vi "ICM Configuration Editor.vi"(11 "Inside a Program?":bool) -> ()   [LabVIEW 2018]
doc: "ICM Configuration Editor.vi\n\nThis Vi is a graphical configuration editor for ICM.\n\nInstrument Communication Module Version 1.0\nJuly, 2017 Original Code Consulting David Thomson\n www.originalcode.com"
uses:
  Controls/ICM Editor Tab.ctl
  Controls/ICM General Parameters.ctl
  Controls/ICM Config Editor State.ctl
  Controls/ICM Editor Command.ctl
  Scaling/Scaling Def.ctl
  Controls/ICM Config Command.ctl
  Query/Query.lvclass
  Scaling/Scaling.lvclass
  Scaling/Scaling.lvclass/Scaling.ctl
  Query/Query.lvclass/Query.ctl
  Query/Write Cycle Time (ms).vi
  Query/Read Cycle Time (ms).vi
  SubVIs/ICM Editor Stop.vi
  Parser/Parser.lvclass
panel:
  in  "File Loaded?":bool
  out "Config File":path
  in  "Stop":bool
  in  "Tab":T1
  in  "Save As":bool
  in  "Open/New":bool
  in  "Save":bool
  in  "Revert":bool
  in  "ICM General Parameters":T2 {"Time" format="%<%H:%M:%S>t"; "Date" format="%<%Y/%m/%d>T"; "Version" format="%.1g"}
  in  "Save Q":bool
  in  "Revert Q":bool
  in  "Cycle Time (ms)":u32
  in  "Queries":u16(ring) items=["Multiple Queries", "No Query", "Single Query"]
  in  "Bus":u16(ring) items=["Clock Time", "Modbus", "NI Analog", "Serial", "UDP"]
  in  "Parser":u16(ring) items=["General Parser", "Multi Sentence Parser", "No-op Parser", "Time Parser"]
  in  "Delete":bool
  in  "Add":bool
  in  "Instance":u16(ring) items=["(none)", "table", "hello", "hi"]
  in  "Save Scaling":bool
  in  "Revert Scaling":bool
  in  "Channel Scalings":i32(listbox)
  in  "Scaling":u16(ring) items=["Lookup Table", "Polynomial"]
  in  "Channel":u16(ring) items=["1", "Hour", "Minute", "Second", "Lat", "Long"]
  out "Error":errorcluster
  in  "Error Continue":bool
  in  "Error Quit":bool
  # "The values for these\nparameters are generally\nset by the ICM system and\nneed not be edited directly."
  # "Entries surrounded by \"***\" are present in the configuration file but\ndo not correspond to existing Channels, Scalings, or Instances."
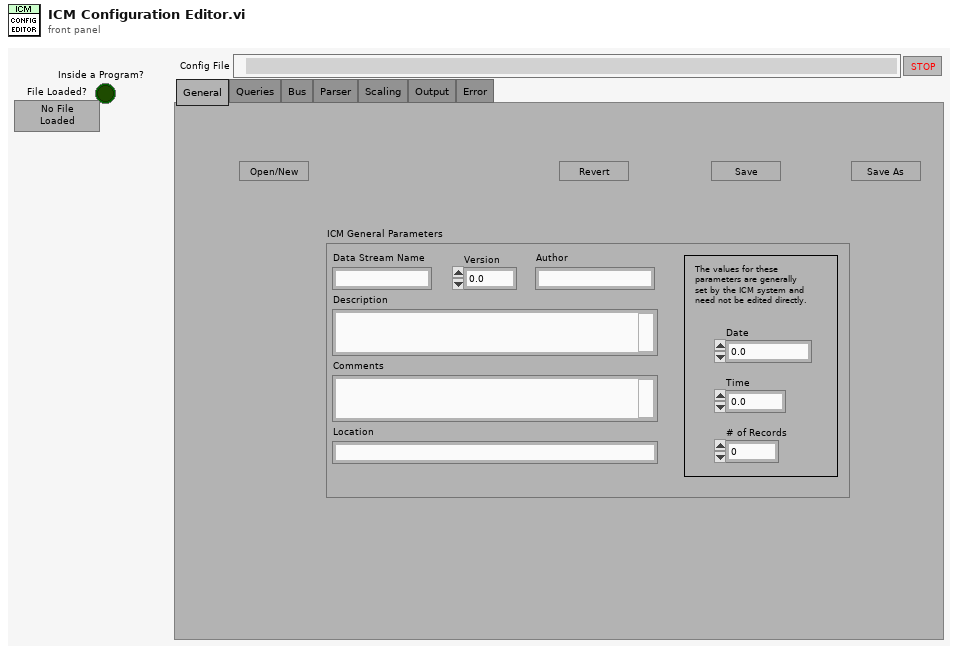
[diagram p1: front panel]
types:
  T1 = typedef "ICM Editor Tab.ctl" = enum32{"General", "Queries", "Bus", "Parser", "Scaling", "Output", "Error"}
  T2 = typedef "ICM General Parameters.ctl" = cluster{"Data Stream Name":string, "Version":sgl, "Author":string, "Description":string, "Comments":string, "Date":dbl, "Time":dbl, "Location":string, "# of Records":i32}
  T3 = typedef "ICM Config Editor State.ctl" = enum16{"Init", "Wait", "Read", "Write", "Load Queries", "Load Bus", "Load Parser", "Display Scaling", "Load Output", "Error", "Stop"}
  T4 = typedef "ICM Config Command.ctl" = enum16{"No-op", "Re-Display Sc."}
  T5 = typedef "ICM Editor Command.ctl" = enum16{"No-op", "Exit"}
  T6 = enum8{"Enabled", "Disabled", "Disabled and Grayed Out"}
  T7 = enum32{"Page Enabled", "Page Disabled", "Page Disabled & Grayed"}
  T8 = typedef "Scaling Def.ctl" = cluster{"Channel":string, "Scaling":string, "Instance":string}
  T9 = cluster{"Query.lvclass":refnum<class "Query.lvclass">, "ICM General Parameters":T2, "Config Queue":refnum<queue>, "Scaling Queue":refnum<queue>, "Query Queue":refnum<queue>, "Parser Queue":refnum<queue>, "Bus Queue":refnum<queue>, "Queries Loaded":bool, "Bus Loaded":bool, "Parser Loaded":bool, "Scaling Loaded":i32, "Instance Loaded":i32, "Scalings":T8[], "Flash?":bool}
  T10 = cluster{"RingText.Text":string, "RingText.Text":string, "RingText.Text":string}
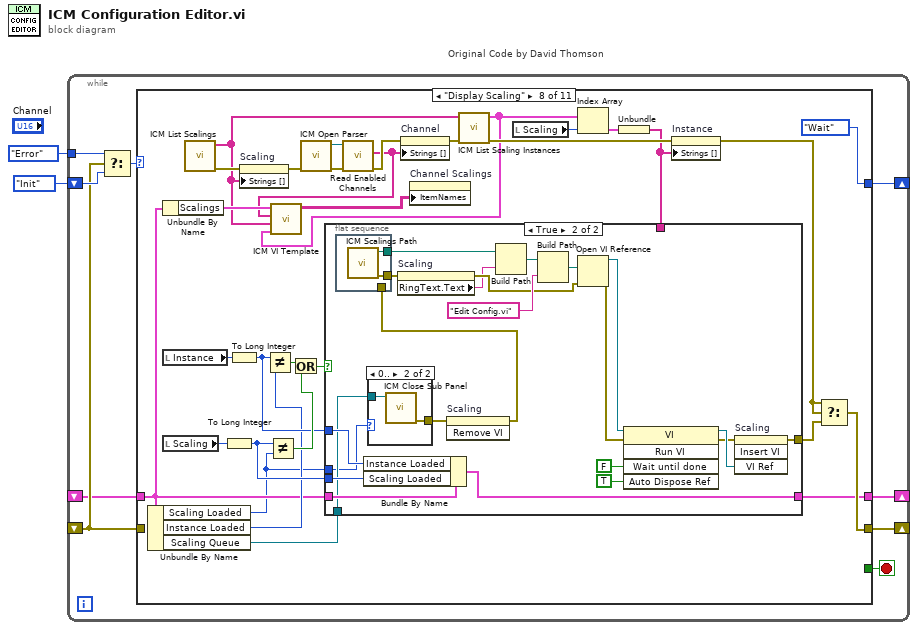
[diagram p0: block diagram]
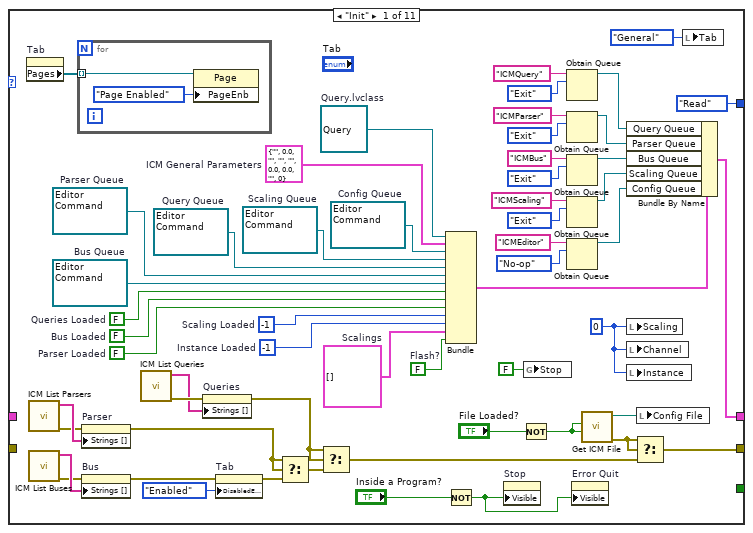
[diagram p2: hidden frame]
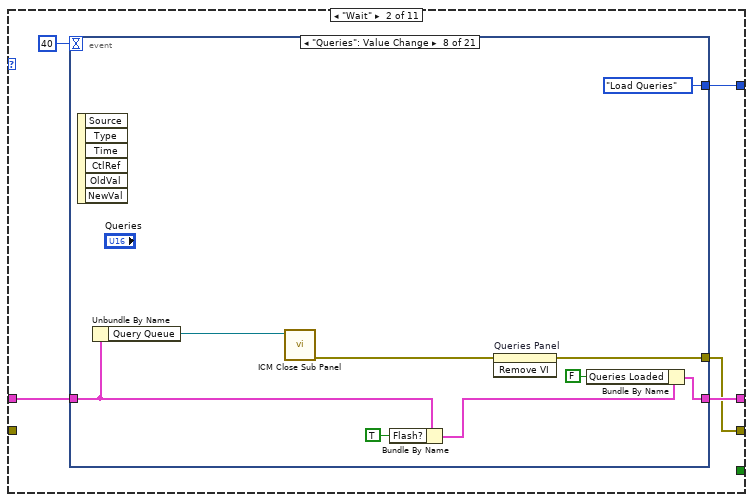
[diagram p3: hidden frame]
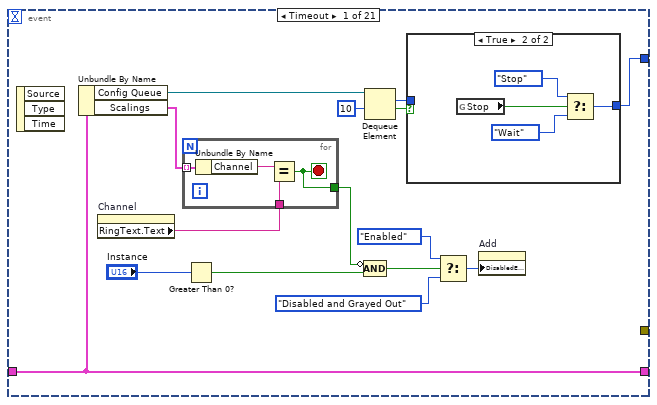
[diagram p4: hidden frame]
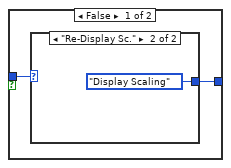
[diagram p5: hidden frame]
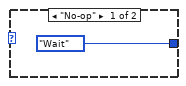
[diagram p6: hidden frame]
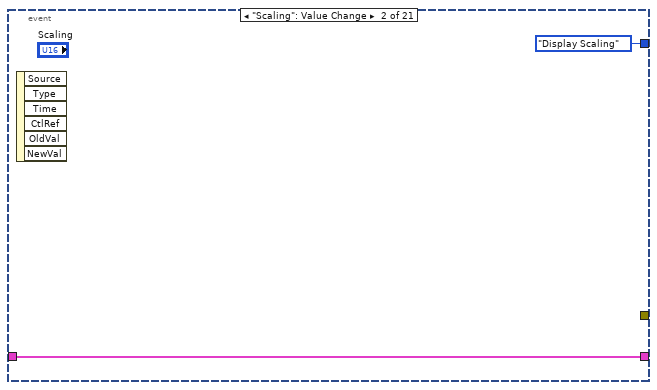
[diagram p7: hidden frame]
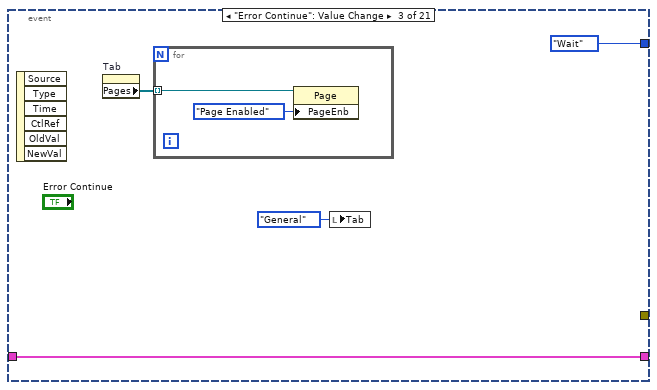
[diagram p8: hidden frame]
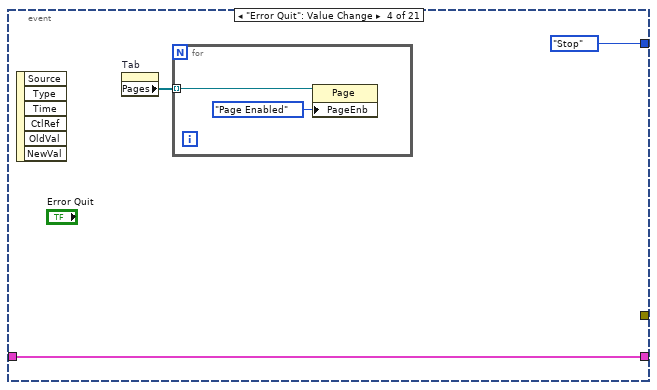
[diagram p9: hidden frame]
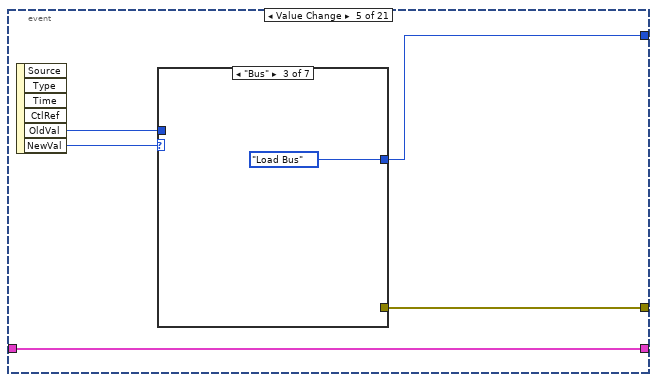
[diagram p10: hidden frame]
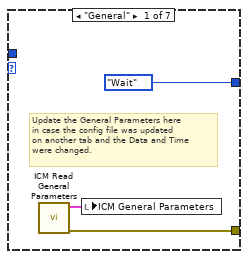
[diagram p11: hidden frame]
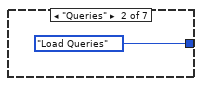
[diagram p12: hidden frame]
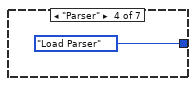
[diagram p13: hidden frame]
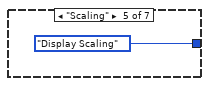
[diagram p14: hidden frame]
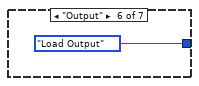
[diagram p15: hidden frame]
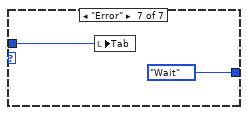
[diagram p16: hidden frame]
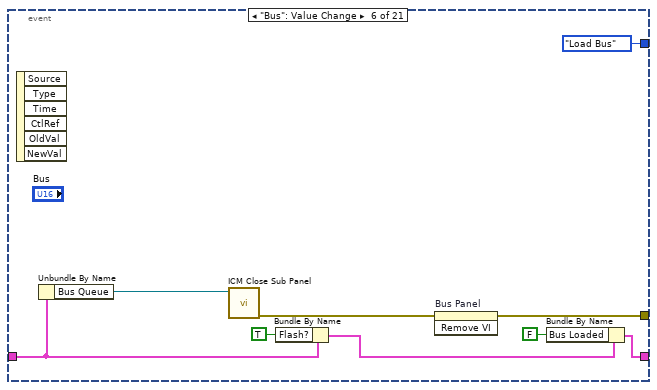
[diagram p17: hidden frame]
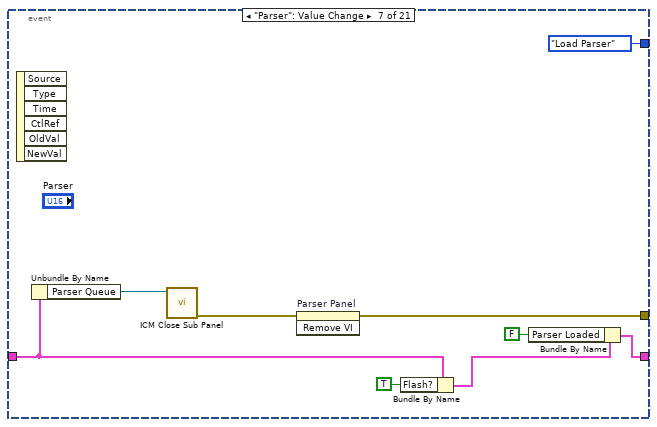
[diagram p18: hidden frame]
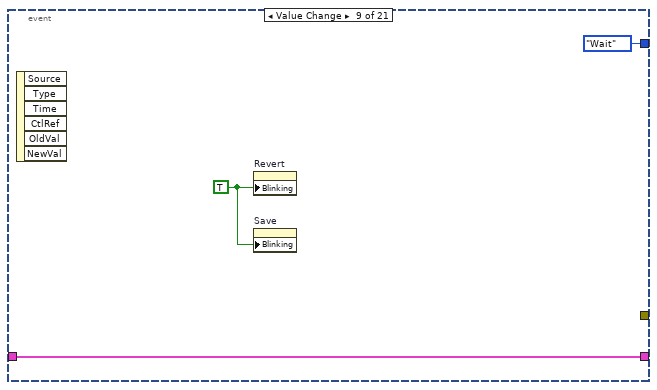
[diagram p19: hidden frame]
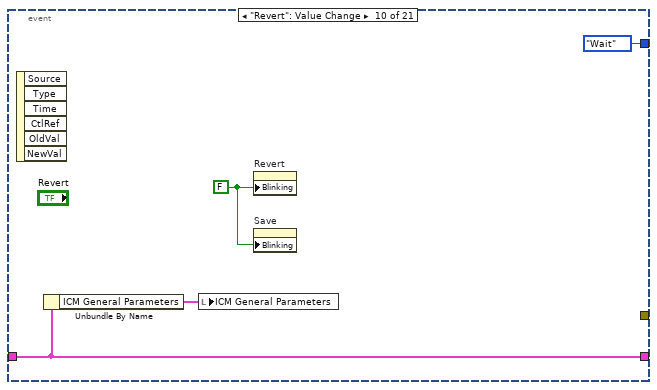
[diagram p20: hidden frame]
diagram:
  n1 = while "Original Code by David Thomson" {
    shift-right: [w5] -> _
    shift-left: ICM_Config_Editor_State."Init" ("Config State") -> [w9]
    shift-right: [w10] -> _
    shift-left: _ -> [w6]
    tunnel: ICM_Config_Editor_State."Error" ("Config State") -> [w7]
    shift-right: [w4] -> _
    shift-left: _ -> [w3]
    stop <- w11 stop-if-true
    n2 = Select(t=w7, s=w6, f=w9) -> (s? t:f=w8:T3)
    n3 = case shown="\"Display Scaling\"" w8 {
      tunnel: [_ _ _ _ _ _ _ _ _ _ TRUE] -> w11
      tunnel: [w60 w70 w261 w288 w297 w332 w361 w412 _ _ _] -> w10
      tunnel: w6 -> [_ _ _ _ _ _ _ _ _ w457 _]
      tunnel: [ICM_Config_Editor_State."Read" ("Config State") w73 ICM_Config_Editor_State."Wait" ("Config State") ICM_Config_Editor_State."Wait" ("Config State") ICM_Config_Editor_State."Wait" ("Config State") ICM_Config_Editor_State."Wait" ("Config State") ICM_Config_Editor_State."Write" ("Config State") ICM_Config_Editor_State."Wait" ("Config State") ICM_Config_Editor_State."Wait" ("Config State") ICM_Config_Editor_State."Wait" ("Config State") ICM_Config_Editor_State."Stop" ("Config State")] -> w5
      tunnel: [w53 w71 w277 w291 w293 w329 w362 w411 w452 w453 w486] -> w4
      tunnel: w3 -> [_ w72 w279 w291 w299 w330 w363 w398 w452 w453 w486]
      frame "Init" {
        w12 = FALSE  # Flash?
        w21 = refnum<class "Query.lvclass"> refnum  # Query.lvclass
        w23 = refnum<queue> refnum items=["No-op", "Re-Display Sc."]  # Config Queue
        w28 = refnum<queue> refnum items=["No-op", "Exit"]  # Scaling Queue
        w31 = u16 0
        w32 = -1  # Instance Loaded
        w34 = -1  # Scaling Loaded
        w33 = T8[] []  # Scalings
        w41 = refnum<queue> refnum items=["No-op", "Exit"]  # Query Queue
        w49 = refnum<queue> refnum items=["No-op", "Exit"]  # Parser Queue
        w50 = FALSE  # Parser Loaded
        w51 = FALSE  # Bus Loaded
        w52 = FALSE  # Queries Loaded
        w56 = refnum<queue> refnum items=["No-op", "Exit"]  # Bus Queue
        w24 = T2 {"Data Stream Name"="", "Version"=0.0, "Author"="", "Description"="", "Comments"="", "Date"=0.0, "Time"=0.0, "Location"="", "# of Records"=0}  # ICM General Parameters
        n4 = property on="Tab" class="TabCtl (strict)"() -> ("Pages"=w59:refnum<vi>[])  [unwired: 2 in, 2 out]
        n5 = call "ICM List Parsers.vi"() -> ("error out"=w45:errorcluster, "Parsers"=w46:string[])  [unwired: 10 in]
        n6 = call "ICM List Buses.vi"() -> ("error out"=w66:errorcluster, "Buses"=w67:string[])  [unwired: 10 in]
        n7 = for {
          tunnel: w59 -> [w69] mode=indexing
          n8 = property class="Page"(reference=w69, "PageEnb"=T7."Page Enabled" ("Page Enabled State")) -> ()  [unwired: 1 in, 2 out]
        }
        n9 = property on="Parser" class="Ring (strict)"(error in=w45, "Strings []"=w46) -> (error out=w43:errorcluster)  [unwired: 1 in, 1 out]
        n10 = property on="Bus" class="Ring (strict)"(error in=w66, "Strings []"=w67) -> (error out=w64:errorcluster)  [unwired: 1 in, 1 out]
        n11 = call "ICM List Queries.vi"() -> ("error out"=w39:errorcluster, "Queries"=w38:string[])  [unwired: 10 in]
        n12 = property on="Queries" class="Ring (strict)"(error in=w39, "Strings []"=w38) -> (error out=w36:errorcluster)  [unwired: 1 in, 1 out]
        n13 = property on="Tab" class="TabCtl (strict)"(error in=w64, "DisabledEnum"=T6."Enabled" ("Disabled")) -> (error out=w44:errorcluster)  [unwired: 1 in, 1 out]
        n14 = Select(t=w43, s=w43, f=w44) -> (s? t:f=w37:errorcluster)
        n15 = Select(t=w36, s=w36, f=w37) -> (s? t:f=w35:errorcluster)
        n16 = Bundle("Query.lvclass"=w21, "ICM General Parameters"=w24, "Config Queue"=w23, "Scaling Queue"=w28, "Query Queue"=w41, "Parser Queue"=w49, "Bus Queue"=w56, "Queries Loaded"=w52, "Bus Loaded"=w51, "Parser Loaded"=w50, "Scaling Loaded"=w34, "Instance Loaded"=w32, "Scalings"=w33, "Flash?"=w12) -> (w55:T9)  [unwired: 1 in]
        n17 = Not(x="Inside a Program?") -> (.not. x?=w14:bool)
        n18 = property on="Stop" class="Bool"("Visible"=w14) -> ()  [unwired: 2 in, 2 out]
        n19 = Not(x="File Loaded?") -> (.not. x?=w16:bool)
        n20 = global write "ICM Editor Stop.vi" "Stop"(FALSE ("Stop")) -> ()
        n21 = Obtain Queue(name (unnamed)="ICMQuery", element data type=ICM_Editor_Command."Exit" ("Editor Command")) -> (queue out=w40:refnum<queue>)  [unwired: 3 in, 2 out]
        n22 = Obtain Queue(name (unnamed)="ICMParser", element data type=ICM_Editor_Command."Exit" ("Editor Command")) -> (queue out=w47:refnum<queue>)  [unwired: 3 in, 2 out]
        n23 = Obtain Queue(name (unnamed)="ICMBus", element data type=ICM_Editor_Command."Exit" ("Editor Command")) -> (queue out=w54:refnum<queue>)  [unwired: 3 in, 2 out]
        n24 = Obtain Queue(name (unnamed)="ICMScaling", element data type=ICM_Editor_Command."Exit" ("Editor Command")) -> (queue out=w27:refnum<queue>)  [unwired: 3 in, 2 out]
        n25 = Obtain Queue(name (unnamed)="ICMEditor", element data type=ICM_Config_Command."No-op" ("Editor Command")) -> (queue out=w22:refnum<queue>)  [unwired: 3 in, 2 out]
        n26 = property on="Error Quit" class="Bool"("Visible"=w14) -> ()  [unwired: 2 in, 2 out]
        n27 = call "Get ICM File.vi"("Re-Init?"=w16, "Allow New?"=w16) -> ("error out"=w61:errorcluster, "ICM File"=w58:path)  [unwired: 8 in]
        n28 = Bundle By Name(cluster=w55, "Query Queue"=w40, "Parser Queue"=w47, "Bus Queue"=w54, "Scaling Queue"=w27, "Config Queue"=w22) -> (w53:T9)
        n29 = local write "Scaling"(w31) -> ()
        n30 = local write "Channel"(w31) -> ()
        n31 = local write "Instance"(w31) -> ()
        n32 = Select(t=w61, s=w61, f=w35) -> (s? t:f=w60:errorcluster)
        n33 = local write "Config File"(w58) -> ()
        n34 = local write "Tab"(ICM_Editor_Tab."General" ("Tab")) -> ()
      }
      frame "Wait" {
        n35 = event shown="[7] \"Queries\": Value Change" {
          selector: _ -> [_ _ _ _ _ _ _ _ _ _ _ _ _ _ _ _ _ _ _ _ _]
          dyn-events: _ -> [_ _ _ _ _ _ _ _ _ _ _ _ _ _ _ _ _ _ _ _ _]
          timeout: 40 -> [_ _ _ _ _ _ _ _ _ _ _ _ _ _ _ _ _ _ _ _ _]
          tunnel: [w85 ICM_Config_Editor_State."Display Scaling" ("Config State") ICM_Config_Editor_State."Wait" ("Config State") ICM_Config_Editor_State."Stop" ("Config State") w118 ICM_Config_Editor_State."Load Bus" ("Config State") ICM_Config_Editor_State."Load Parser" ("Config State") ICM_Config_Editor_State."Load Queries" ("Config State") ICM_Config_Editor_State."Wait" ("Config State") ICM_Config_Editor_State."Wait" ("Config State") ICM_Config_Editor_State."Write" ("Config State") ICM_Config_Editor_State."Read" ("Config State") w186 ICM_Config_Editor_State."Stop" ("Config State") ICM_Config_Editor_State."Display Scaling" ("Config State") ICM_Config_Editor_State."Display Scaling" ("Config State") ICM_Config_Editor_State."Wait" ("Config State") ICM_Config_Editor_State."Display Scaling" ("Config State") ICM_Config_Editor_State."Wait" ("Config State") ICM_Config_Editor_State."Wait" ("Config State") ICM_Config_Editor_State."Wait" ("Config State")] -> w73
          tunnel: w72 -> [w89 w103 w104 w110 w117 w131 w139 w148 w157 w161 w166 w171 w177 w200 w206 w222 w231 w236 w243 w252 w255]
          tunnel: [w89 w103 w104 w110 w117 w136 w146 w155 w157 w161 w164 w171 w185 w200 w205 w221 w231 w235 w243 w252 w255] -> w71
          tunnel: [_ _ _ _ w116 w137 w144 w153 _ _ _ _ w176 _ _ _ w227 w234 _ w247 w253] -> w70
          event Timeout {
            n36 = event-data() -> ()  [unwired: 1 in, 3 out]
            n37 = Unbundle By Name(w89) -> ("Config Queue"=w88:refnum<queue>, "Scalings"=w83:T8[])
            n38 = property on="Channel" class="Ring (strict)"() -> ("RingText.Text"=w82:string)  [unwired: 2 in, 2 out]
            n39 = for {
              tunnel: w83 -> [w91] mode=indexing
              tunnel: [w93] -> w81
              tunnel: w82 -> [w90]
              stop <- w93 stop-if-true
              n40 = Unbundle By Name(w91) -> ("Channel"=w92:string)
              n41 = Equal?(x=w92, y=w90) -> (x = y?=w93:bool)
            }
            n42 = Greater Than 0?(x="Instance") -> (x > 0?=w79:bool)
            n43 = Compound Arithmetic op=AND(invert w81, w79) -> (w76:bool)
            n44 = Dequeue Element(queue=w88, timeout in ms (-1)=10) -> (element=w84:T4, timed out?=w86:bool)  [unwired: 1 in, 2 out]
            n45 = case shown="True" w86 {
              tunnel: [w94 w101] -> w85
              tunnel: w84 -> [w95 _]
              frame False {
                n46 = case shown="\"Re-Display Sc.\"" w95 {
                  tunnel: [ICM_Config_Editor_State."Wait" ("Config State") ICM_Config_Editor_State."Display Scaling" ("Config State")] -> w94
                  frame "No-op" {
                  }
                  frame "Re-Display Sc." {
                  }
                }
              }
              frame True {
                n47 = global read "ICM Editor Stop.vi" "Stop"() -> (w100:bool)
                n48 = Select(t=ICM_Config_Editor_State."Stop" ("Config State"), s=w100, f=ICM_Config_Editor_State."Wait" ("Config State")) -> (s? t:f=w101:T3)
              }
            }
            n49 = Select(t=T6."Enabled" ("Disabled"), s=w76, f=T6."Disabled and Grayed Out" ("Disabled")) -> (s? t:f=w75:T6)
            n50 = property on="Add" class="Bool"("DisabledEnum"=w75) -> ()  [unwired: 2 in, 2 out]
          }
          event "Scaling": Value Change {
            n51 = event-data() -> ()  [unwired: 1 in, 6 out]
          }
          event "Error Continue": Value Change {
            n52 = event-data() -> ()  [unwired: 1 in, 6 out]
            n53 = property on="Tab" class="TabCtl (strict)"() -> ("Pages"=w105:refnum<vi>[])  [unwired: 2 in, 2 out]
            n54 = for {
              tunnel: w105 -> [w109] mode=indexing
              n55 = property class="Page"(reference=w109, "PageEnb"=T7."Page Enabled" ("Page Enabled State")) -> ()  [unwired: 1 in, 2 out]
            }
            n56 = local write "Tab"(ICM_Editor_Tab."General" ("Tab")) -> ()
          }
          event "Error Quit": Value Change {
            n57 = event-data() -> ()  [unwired: 1 in, 6 out]
            n58 = property on="Tab" class="TabCtl (strict)"() -> ("Pages"=w111:refnum<vi>[])  [unwired: 2 in, 2 out]
            n59 = for {
              tunnel: w111 -> [w114] mode=indexing
              n60 = property class="Page"(reference=w114, "PageEnb"=T7."Page Enabled" ("Page Enabled State")) -> ()  [unwired: 1 in, 2 out]
            }
          }
          event Value Change {
            n61 = event-data() -> ("OldVal"=w115:T1, "NewVal"=w119:T1)  [unwired: 1 in, 4 out]
            n62 = case shown="\"Bus\"" w119 {
              tunnel: [ICM_Config_Editor_State."Wait" ("Config State") ICM_Config_Editor_State."Load Queries" ("Config State") ICM_Config_Editor_State."Load Bus" ("Config State") ICM_Config_Editor_State."Load Parser" ("Config State") ICM_Config_Editor_State."Display Scaling" ("Config State") ICM_Config_Editor_State."Load Output" ("Config State") ICM_Config_Editor_State."Wait" ("Config State")] -> w118
              tunnel: [w120 _ _ _ _ _ _] -> w116
              tunnel: w115 -> [_ _ _ _ _ _ w128]
              frame "General" {
                # "Update the General Parameters here\nin case the config file was updated\non another tab and the Data and Time\nwere changed."
                n63 = call "ICM Read General Parameters.vi"() -> ("error out"=w120:errorcluster, "ICM General Parameters"=w121:T2)  [unwired: 7 in, 3 out]
                n64 = local write "ICM General Parameters"(w121) -> ()
              }
              frame "Queries" {
              }
              frame "Bus" {
              }
              frame "Parser" {
              }
              frame "Scaling" {
              }
              frame "Output" {
              }
              frame "Error" {
                n65 = local write "Tab"(w128) -> ()
              }
            }
          }
          event "Bus": Value Change {
            n66 = event-data() -> ()  [unwired: 1 in, 6 out]
            n67 = Unbundle By Name(w131) -> ("Bus Queue"=w134:refnum<queue>)
            n68 = call "ICM Close Sub Panel.vi"("Queue"=w134) -> ("error out"=w133:errorcluster)  [unwired: 9 in, 1 out]
            n69 = Bundle By Name(cluster=w131, "Flash?"=TRUE) -> (w132:T9)
            n70 = invoke on="Bus Panel" class="SubPnl" method="Remove VI"(error in=w133) -> (error out=w137:errorcluster)  [unwired: 2 in, 2 out]
            n71 = Bundle By Name(cluster=w132, "Bus Loaded"=FALSE) -> (w136:T9)
          }
          event "Parser": Value Change {
            n72 = event-data() -> ()  [unwired: 1 in, 6 out]
            n73 = Unbundle By Name(w139) -> ("Parser Queue"=w143:refnum<queue>)
            n74 = call "ICM Close Sub Panel.vi"("Queue"=w143) -> ("error out"=w142:errorcluster)  [unwired: 9 in, 1 out]
            n75 = invoke on="Parser Panel" class="SubPnl" method="Remove VI"(error in=w142) -> (error out=w144:errorcluster)  [unwired: 2 in, 2 out]
            n76 = Bundle By Name(cluster=w139, "Flash?"=TRUE) -> (w140:T9)
            n77 = Bundle By Name(cluster=w140, "Parser Loaded"=FALSE ("Bus Loaded")) -> (w146:T9)
          }
          event "Queries": Value Change {
            n78 = event-data() -> ()  [unwired: 1 in, 6 out]
            n79 = Unbundle By Name(w148) -> ("Query Queue"=w152:refnum<queue>)
            n80 = call "ICM Close Sub Panel.vi"("Queue"=w152) -> ("error out"=w151:errorcluster)  [unwired: 9 in, 1 out]
            n81 = Bundle By Name(cluster=w148, "Flash?"=TRUE) -> (w149:T9)
            n82 = invoke on="Queries Panel" class="SubPnl" method="Remove VI"(error in=w151) -> (error out=w153:errorcluster)  [unwired: 2 in, 2 out]
            n83 = Bundle By Name(cluster=w149, "Queries Loaded"=FALSE ("Bus Loaded")) -> (w155:T9)
          }
          event Value Change {
            w159 = TRUE ("Blinking")
            n84 = event-data() -> ()  [unwired: 1 in, 6 out]
            n85 = property on="Revert" class="Bool"("Blinking"=w159) -> ()  [unwired: 2 in, 2 out]
            n86 = property on="Save" class="Bool"("Blinking"=w159) -> ()  [unwired: 2 in, 2 out]
          }
          event "Revert": Value Change {
            w163 = FALSE ("Blinking")
            n87 = event-data() -> ()  [unwired: 1 in, 6 out]
            n88 = Unbundle By Name(w161) -> ("ICM General Parameters"=w160:T2)
            n89 = local write "ICM General Parameters"(w160) -> ()
            n90 = property on="Revert" class="Bool"("Blinking"=w163) -> ()  [unwired: 2 in, 2 out]
            n91 = property on="Save" class="Bool"("Blinking"=w163) -> ()  [unwired: 2 in, 2 out]
          }
          event "Save": Value Change {
            w168 = FALSE ("Blinking")
            n92 = event-data() -> ()  [unwired: 1 in, 6 out]
            n93 = property on="Revert" class="Bool"("Blinking"=w168) -> ()  [unwired: 2 in, 2 out]
            n94 = property on="Save" class="Bool"("Blinking"=w168) -> ()  [unwired: 2 in, 2 out]
            n95 = Bundle By Name(cluster=w166, "ICM General Parameters"="ICM General Parameters") -> (w164:T9)
          }
          event "Open/New": Value Change {
            w169 = TRUE ("Re-Init?")
            n96 = event-data() -> ()  [unwired: 1 in, 6 out]
            n97 = call "Get ICM File.vi"("Re-Init?"=w169, "Allow New?"=w169) -> ("ICM File"=→"Config File":path)  [unwired: 8 in, 1 out]
          }
          event "Save As": Value Change {
            n98 = event-data() -> ()  [unwired: 1 in, 6 out]
            n99 = call "Get ICM File.vi"() -> ("error out"=w179:errorcluster, "ICM File"=w178:path)  [unwired: 10 in]
            n100 = Strip Path(path=w178) -> (stripped path=w184:path)  [unwired: 1 out]
            n101 = call "File Dialog"("start path"=w184, "prompt"="Name the new configuration file:" ("pattern label"), "error in"=w179, "pattern (all files)"=".icm", "pattern label"="ICM Configuraiton File") -> ("selected path"=w180:path, "cancelled"=w174:bool, "error out"=w175:errorcluster)  [unwired: 7 in, 1 out]
            n102 = Compound Arithmetic op=AND(invert w174, invert w175) -> (w173:bool)
            n103 = case shown="True" w173 {
              tunnel: [ICM_Config_Editor_State."Wait" ("Config State") ICM_Config_Editor_State."Write" ("Config State")] -> w186
              tunnel: [w188 w190] -> w185
              tunnel: w180 -> [_ w195]
              tunnel: w178 -> [_ w197]
              tunnel: w177 -> [w188 w191]
              tunnel: [_ w192] -> w176
              frame False {
              }
              frame True {
                w198 = FALSE ("Blinking")
                n104 = Copy(9:TRUE ("overwrite (F)"), 10:w195, 11:w197) -> (0:w193:errorcluster)  [unwired: 2 in, 2 out]
                n105 = call "Get ICM File.vi"("ICM File In"=w195) -> ("error out"=w194:errorcluster)  [unwired: 9 in, 1 out]
                n106 = Select(t=w194, s=w194, f=w193) -> (s? t:f=w192:errorcluster)
                n107 = local read "ICM General Parameters"() -> (w189:T2)
                n108 = Bundle By Name(cluster=w191, "ICM General Parameters"=w189) -> (w190:T9)
                n109 = property on="Revert" class="Bool"("Blinking"=w198) -> ()  [unwired: 2 in, 2 out]
                n110 = property on="Save" class="Bool"("Blinking"=w198) -> ()  [unwired: 2 in, 2 out]
              }
            }
          }
          event "Stop": Value Change {
            n111 = event-data() -> ()  [unwired: 1 in, 6 out]
          }
          event "Add": Value Change {
            n112 = event-data() -> ()  [unwired: 1 in, 6 out]
            n113 = property on="Channel" class="Ring (strict)"() -> ("RingText.Text"=w204:string)  [unwired: 2 in, 2 out]
            n114 = property on="Scaling" class="Ring (strict)"() -> ("RingText.Text"=w210:string)  [unwired: 2 in, 2 out]
            n115 = property on="Instance" class="Ring (strict)"() -> ("RingText.Text"=w209:string)  [unwired: 2 in, 2 out]
            n116 = Unbundle By Name(w206) -> ("Scalings"=w203:T8[])
            n117 = Bundle("RingText.Text"=w204, "RingText.Text"=w210, "RingText.Text"=w209) -> (w208:T10)  [unwired: 1 in]
            n118 = for {
              tunnel: w204 -> [w213]
              tunnel: w203 -> [w215] mode=indexing
              tunnel: [w212] -> w202
              stop <- w212 stop-if-true
              n119 = Unbundle By Name(w215) -> ("Channel"=w214:string)
              n120 = Equal?(x=w213, y=w214) -> (x = y?=w212:bool)
            }
            n121 = case shown="False" w202 {
              tunnel: w208 -> [w218 _]
              tunnel: w203 -> [w217 w219]
              tunnel: [w216 w219] -> w207
              frame False {
                n122 = Build Array (concatenate)(w218, w217) -> (w216:T8[])
              }
              frame True {
              }
            }
            n123 = Bundle By Name(cluster=w206, "Scalings"=w207) -> (w205:T9)
          }
          event "Delete": Value Change {
            n124 = event-data() -> ()  [unwired: 1 in, 6 out]
            n125 = Unbundle By Name(w222) -> ("Scalings"=w225:T8[])
            n126 = Delete From Array(array=w225, length=1, index="Channel Scalings") -> (array with subset deleted=w223:T8[])  [unwired: 1 out]
            n127 = Bundle By Name(cluster=w222, "Scalings"=w223) -> (w221:T9)
          }
          event "Save Scaling": Value Change {
            n128 = event-data() -> ()  [unwired: 1 in, 6 out]
            n129 = Unbundle By Name(w231) -> ("Scalings"=w230:T8[])
            n130 = call "Write Scalings.vi"("Scalings"=w230, "Scaling in"=refnum<class "Scaling.lvclass"> refnum ("Scaling.lvclass")) -> ("error out"=w228:errorcluster, "Scaling out"=w229:refnum<class "Scaling.lvclass">)  [unwired: 8 in]
            n131 = call-dynamic "Write Config.vi"("error in (no error)"=w228, "Scaling in"=w229) -> ("error out"=w227:errorcluster)  [unwired: 8 in, 1 out]
          }
          event "Revert Scaling": Value Change {
            n132 = event-data() -> ()  [unwired: 1 in, 6 out]
            n133 = call-dynamic "Read Config.vi"("Scaling in"=refnum<class "Scaling.lvclass"> refnum ("Scaling.lvclass")) -> ("error out"=w239:errorcluster, "Scaling out"=w238:refnum<class "Scaling.lvclass">)  [unwired: 9 in]
            n134 = call "Read Scalings.vi"("error in (no error)"=w239, "Scaling in"=w238) -> ("error out"=w234:errorcluster, "Scalings"=w237:T8[])  [unwired: 7 in, 1 out]
            n135 = Bundle By Name(cluster=w236, "Scalings"=w237) -> (w235:T9)
          }
          event "Cycle Time (ms)": Value Change {
            w242 = TRUE ("Blinking")
            n136 = event-data() -> ()  [unwired: 1 in, 6 out]
            n137 = property on="Revert Q" class="Bool"("Blinking"=w242) -> ()  [unwired: 2 in, 2 out]
            n138 = property on="Save Q" class="Bool"("Blinking"=w242) -> ()  [unwired: 2 in, 2 out]
          }
          event "Save Q": Value Change {
            w245 = FALSE ("Blinking")
            n139 = event-data() -> ()  [unwired: 1 in, 6 out]
            n140 = Unbundle By Name(w252) -> ("Query.lvclass"=w251:refnum<class "Query.lvclass">)
            n141 = property class="Query.lvclass"(reference=w251, "Properties:Cycle Time (ms)"="Cycle Time (ms)") -> (reference out=w249:refnum<class "Query.lvclass">, error out=w248:errorcluster)  [unwired: 1 in]
            n142 = call-dynamic "Write Config.vi"("error in (no error)"=w248, "Query in"=w249) -> ("error out"=w247:errorcluster)  [unwired: 8 in, 1 out]
            n143 = property on="Revert Q" class="Bool"("Blinking"=w245) -> ()  [unwired: 2 in, 2 out]
            n144 = property on="Save Q" class="Bool"("Blinking"=w245) -> ()  [unwired: 2 in, 2 out]
          }
          event "Revert Q": Value Change {
            w258 = FALSE ("Blinking")
            n145 = event-data() -> ()  [unwired: 1 in, 6 out]
            n146 = property on="Revert Q" class="Bool"("Blinking"=w258) -> ()  [unwired: 2 in, 2 out]
            n147 = property on="Save Q" class="Bool"("Blinking"=w258) -> ()  [unwired: 2 in, 2 out]
            n148 = Unbundle By Name(w255) -> ("Query.lvclass"=w256:refnum<class "Query.lvclass">)
            n149 = property class="Query.lvclass"(reference=w256) -> (error out=w253:errorcluster, "Properties:Cycle Time (ms)"=w254:u32)  [unwired: 1 in, 1 out]
            n150 = local write "Cycle Time (ms)"(w254) -> ()
          }
        }
      }
      frame "Read" {
        n151 = property on="Queries" class="Ring (strict)"() -> ("Strings []"=w267:string[])  [unwired: 2 in, 2 out]
        n152 = property on="Bus" class="Ring (strict)"() -> ("Strings []"=w284:string[])  [unwired: 2 in, 2 out]
        n153 = property on="Parser" class="Ring (strict)"() -> ("Strings []"=w271:string[])  [unwired: 2 in, 2 out]
        n154 = call "ICM Read General Parameters.vi"() -> ("error out"=w264:errorcluster, "Parser"=w273:string, "Bus"=w285:string, "ICM General Parameters"=w278:T2, "Query"=w265:string)  [unwired: 7 in]
        n155 = Search 1D Array(1D array=w284, element=w285) -> (index of element=w282:i32)  [unwired: 1 in]
        n156 = Search 1D Array(1D array=w271, element=w273) -> (index of element=w275:i32)  [unwired: 1 in]
        n157 = Search 1D Array(1D array=w267, element=w265) -> (index of element=w270:i32)  [unwired: 1 in]
        n158 = Less Than 0?(x=w282) -> (x < 0?=w283:bool)
        n159 = Less Than 0?(x=w275) -> (x < 0?=w274:bool)
        n160 = Less Than 0?(x=w270) -> (x < 0?=w269:bool)
        n161 = call-dynamic "Read Config.vi"("error in (no error)"=w264, "Scaling in"=refnum<class "Scaling.lvclass"> refnum ("Scaling.lvclass")) -> ("error out"=w262:errorcluster, "Scaling out"=w260:refnum<class "Scaling.lvclass">)  [unwired: 8 in]
        n162 = Select(t=0, s=w283, f=w282) -> (s? t:f=w280:i32)
        n163 = Select(t=0, s=w274, f=w275) -> (s? t:f=w272:i32)
        n164 = Select(t=0, s=w269, f=w270) -> (s? t:f=w266:i32)
        n165 = local write "Queries"(w266) -> ()
        n166 = local write "Bus"(w280) -> ()
        n167 = local write "Parser"(w272) -> ()
        n168 = call "Read Scalings.vi"("error in (no error)"=w262, "Scaling in"=w260) -> ("error out"=w261:errorcluster, "Scalings"=w259:T8[])  [unwired: 7 in, 1 out]
        n169 = local write "ICM General Parameters"(w278) -> ()
        n170 = Bundle By Name(cluster=w279, "ICM General Parameters"=w278, "Scalings"=w259) -> (w277:T9)
      }
      frame "Write" {
        n171 = Unbundle By Name(w291) -> ("ICM General Parameters"=w290:T2)
        n172 = call "ICM Write General Parameters.vi"("ICM General Parameters"=w290) -> ("error out"=w289:errorcluster)  [unwired: 10 in]
        n173 = call "ICM Update Date and Time.vi"("error in (no error)"=w289) -> ("error out"=w288:errorcluster, "output cluster"=w287:T2)  [unwired: 9 in]
        n174 = local write "ICM General Parameters"(w287) -> ()
      }
      frame "Load Queries" {
        n175 = Unbundle By Name(w299) -> ("Query.lvclass"=w298:refnum<class "Query.lvclass">, "Queries Loaded"=w300:bool)
        n176 = call-dynamic "Read Config.vi"("Query in"=w298) -> ("error out"=w295:errorcluster, "Query out"=w296:refnum<class "Query.lvclass">)  [unwired: 9 in]
        n177 = case shown="False" w300 {
          tunnel: [w313 _] -> w297
          tunnel: w299 -> [w302 w328]
          tunnel: [w314 w328] -> w293
          frame False {
            n178 = call "ICM Queries Path.vi"() -> ("error out"=w308:errorcluster, "ICM Queries Path"=w322:path)  [unwired: 10 in]
            n179 = property on="Queries" class="Ring (strict)"(error in=w308) -> (error out=w309:errorcluster, "RingText.Text"=w310:string)  [unwired: 1 in, 1 out]
            n180 = Unbundle By Name(w302) -> ("Flash?"=w307:bool)
            n181 = Build Path(base path=w322, name or relative path=w310) -> (appended path=w321:path)
            n182 = Build Path(base path=w321, name or relative path="Edit Config.vi") -> (appended path=w319:path)
            n183 = Open VI Reference(vi path=w319, error in (no error)=w309) -> (vi reference=w305:refnum<vi>, error out=w318:errorcluster)  [unwired: 4 in]
            n184 = case shown="True" w307 {
              tunnel: w305 -> [w323 w325]
              tunnel: [w323 w324] -> w304
              frame False {
              }
              frame True {
                n185 = invoke class="VI" method="Ctrl Val.Set"(reference=w325, "Control Name"="Flash Save", "Value"=TRUE ("Bus Loaded")) -> (reference out=w324:refnum<vi>)  [unwired: 2 in, 4 out]
              }
            }
            n186 = Bundle By Name(cluster=w302, "Flash?"=FALSE) -> (w303:T9)
            n187 = invoke class="VI" method="Run VI"(reference=w304, error in=w318, "Wait until done"=FALSE ("Wait Until Done"), "Auto Dispose Ref"=TRUE ("Auto Dispose Reference")) -> (reference out=w311:refnum<vi>, error out=w312:errorcluster)  [unwired: 1 in, 3 out]
            n188 = Bundle By Name(cluster=w303, "Queries Loaded"=TRUE ("Bus Loaded")) -> (w314:T9)
            n189 = invoke on="Queries Panel" class="SubPnl" method="Insert VI"(error in=w312, "VI Ref"=w311) -> (error out=w313:errorcluster)  [unwired: 2 in, 3 out]
          }
          frame True {
          }
        }
        n190 = property class="Query.lvclass"(reference=w296, error in=w295) -> ("Properties:Cycle Time (ms)"=w294:u32)  [unwired: 2 out]
        n191 = local write "Cycle Time (ms)"(w294) -> ()
      }
      frame "Load Bus" {
        n192 = Unbundle By Name(w330) -> ("Bus Loaded"=w331:bool)
        n193 = case shown="False" w331 {
          tunnel: [w342 _] -> w332
          tunnel: w330 -> [w335 w360]
          tunnel: [w340 w360] -> w329
          frame False {
            n194 = call "ICM Buses Path.vi"() -> ("error out"=w354:errorcluster, "ICM Buses Path"=w353:path)  [unwired: 10 in]
            n195 = property on="Bus" class="Ring (strict)"(error in=w354) -> (error out=w347:errorcluster, "RingText.Text"=w352:string)  [unwired: 1 in, 1 out]
            n196 = Build Path(base path=w353, name or relative path=w352) -> (appended path=w351:path)
            n197 = Unbundle By Name(w335) -> ("Flash?"=w337:bool)
            n198 = Build Path(base path=w351, name or relative path="Edit Config.vi") -> (appended path=w349:path)
            n199 = Open VI Reference(vi path=w349, error in (no error)=w347) -> (vi reference=w339:refnum<vi>, error out=w348:errorcluster)  [unwired: 4 in]
            n200 = case shown="True" w337 {
              tunnel: w339 -> [w355 w357]
              tunnel: [w355 w356] -> w338
              frame False {
              }
              frame True {
                n201 = invoke class="VI" method="Ctrl Val.Set"(reference=w357, "Control Name"="Flash Save", "Value"=TRUE ("Bus Loaded")) -> (reference out=w356:refnum<vi>)  [unwired: 2 in, 4 out]
              }
            }
            n202 = Bundle By Name(cluster=w335, "Flash?"=FALSE) -> (w336:T9)
            n203 = invoke class="VI" method="Run VI"(reference=w338, error in=w348, "Wait until done"=FALSE ("Wait Until Done"), "Auto Dispose Ref"=TRUE ("Auto Dispose Reference")) -> (reference out=w343:refnum<vi>, error out=w344:errorcluster)  [unwired: 1 in, 3 out]
            n204 = Bundle By Name(cluster=w336, "Bus Loaded"=TRUE) -> (w340:T9)
            n205 = invoke on="Bus Panel" class="SubPnl" method="Insert VI"(error in=w344, "VI Ref"=w343) -> (error out=w342:errorcluster)  [unwired: 2 in, 3 out]
          }
          frame True {
          }
        }
      }
      frame "Load Parser" {
        n206 = Unbundle By Name(w363) -> ("Parser Loaded"=w364:bool)
        n207 = case shown="False" w364 {
          tunnel: [w377 _] -> w361
          tunnel: w363 -> [w369 w392]
          tunnel: [w378 w392] -> w362
          frame False {
            n208 = call "ICM Parsers Path.vi"() -> ("error out"=w373:errorcluster, "ICM Parsers Path"=w386:path)  [unwired: 10 in]
            n209 = property on="Parser" class="Ring (strict)"(error in=w373) -> (error out=w372:errorcluster, "RingText.Text"=w374:string)  [unwired: 1 in, 1 out]
            n210 = Unbundle By Name(w369) -> ("Flash?"=w371:bool)
            n211 = Build Path(base path=w386, name or relative path=w374) -> (appended path=w385:path)
            n212 = Build Path(base path=w385, name or relative path="Edit Config.vi") -> (appended path=w383:path)
            n213 = Open VI Reference(vi path=w383, error in (no error)=w372) -> (vi reference=w367:refnum<vi>, error out=w382:errorcluster)  [unwired: 4 in]
            n214 = case shown="True" w371 {
              tunnel: w367 -> [w387 w389]
              tunnel: [w387 w388] -> w366
              frame False {
              }
              frame True {
                n215 = invoke class="VI" method="Ctrl Val.Set"(reference=w389, "Control Name"="Flash Save", "Value"=TRUE ("Bus Loaded")) -> (reference out=w388:refnum<vi>)  [unwired: 2 in, 4 out]
              }
            }
            n216 = Bundle By Name(cluster=w369, "Flash?"=FALSE) -> (w368:T9)
            n217 = invoke class="VI" method="Run VI"(reference=w366, error in=w382, "Wait until done"=FALSE ("Wait Until Done"), "Auto Dispose Ref"=TRUE ("Auto Dispose Reference")) -> (reference out=w375:refnum<vi>, error out=w376:errorcluster)  [unwired: 1 in, 3 out]
            n218 = Bundle By Name(cluster=w368, "Parser Loaded"=TRUE ("Bus Loaded")) -> (w378:T9)
            n219 = invoke on="Parser Panel" class="SubPnl" method="Insert VI"(error in=w376, "VI Ref"=w375) -> (error out=w377:errorcluster)  [unwired: 2 in, 3 out]
          }
          frame True {
          }
        }
      }
      frame "Display Scaling" {
        n220 = Unbundle By Name(w398) -> ("Scaling Loaded"=w393:i32, "Instance Loaded"=w403:i32, "Scaling Queue"=w402:refnum<queue>)
        n221 = Unbundle By Name(w398) -> ("Scalings"=w397:T8[])
        n222 = local read "Instance"() -> (w409:u16)
        n223 = local read "Scaling"() -> (w410:u16)
        n224 = call "ICM List Scalings.vi"() -> ("error out"=w419:errorcluster, "Scalings"=w396:string[])  [unwired: 10 in]
        n225 = To Long Integer(number=w410) -> (32bit integer=w406:i32)
        n226 = To Long Integer(number=w409) -> (32bit integer=w404:i32)
        n227 = property on="Scaling" class="Ring (strict)"(error in=w419, "Strings []"=w396) -> (error out=w418:errorcluster)  [unwired: 1 in, 1 out]
        n228 = Not Equal?(x=w404, y=w403) -> (x != y?=w407:bool)
        n229 = Not Equal?(x=w406, y=w393) -> (x != y?=w405:bool)
        n230 = Or(x=w407, y=w405) -> (x .or. y?=w408:bool)
        n231 = call "ICM Open Parser.vi"("error in (no error)"=w418) -> ("error out"=w421:errorcluster, "Parser out"=w422:refnum<class "Parser.lvclass">)  [unwired: 9 in]
        n232 = call-dynamic "Read Enabled Channels.vi"("error in (no error)"=w421, "Parser in"=w422) -> ("error out"=w420:errorcluster, "Enabled Channels"=w395:string[])  [unwired: 7 in, 1 out]
        n233 = property on="Channel" class="Ring (strict)"(error in=w420, "Strings []"=w395) -> (error out=w417:errorcluster)  [unwired: 1 in, 1 out]
        n234 = call "ICM List Scaling Instances.vi"("error in (no error)"=w417, "Scalings"=w396) -> ("error out"=w416:errorcluster, "Instances"=w394:cluster{"Instances":string[]}[])  [unwired: 8 in]
        n235 = call "ICM VI Template.vi"("Instances"=w394, "Scalings"=w396, "Channels"=w395, "Scalings In"=w397) -> ("Table"=w399:string[][])  [unwired: 7 in]
        n236 = property on="Channel Scalings" class="MCListbox (strict)"("ItemNames"=w399) -> ()  [unwired: 2 in, 2 out]
        n237 = local read "Scaling"() -> (w414:u16)
        n238 = Index Array(array=w394, index=w414) -> (element=w415:cluster{"Instances":string[]})
        n239 = Unbundle(w415) -> ("Instances"=w400:string[])
        n240 = case shown="True" w408 {
          tunnel: [_ w435] -> w413
          tunnel: w398 -> [w424 w434]
          tunnel: [w424 w433] -> w411
          tunnel: w406 -> [_ w432]
          tunnel: w404 -> [_ w431]
          tunnel: w402 -> [_ w430]
          tunnel: w400 -> [_ _]
          tunnel: w393 -> [_ w427]
          frame False {
          }
          frame True {
            n241 = flat-sequence {
              tunnel: [w450] -> w446
              tunnel: [w449] -> w438
              tunnel: w428 -> [_]
              frame #0 {
                n242 = call "ICM Scalings Path.vi"() -> ("error out"=w449:errorcluster, "ICM Scalings Path"=w450:path)  [unwired: 10 in]
              }
            }
            n243 = Bundle By Name(cluster=w434, "Instance Loaded"=w431, "Scaling Loaded"=w432) -> (w433:T9)
            n244 = case shown="0.." w427 {
              tunnel: w430 -> [_ w448]
              tunnel: [_ w447] -> w429
              frame ..-1 {
              }
              frame 0.. {
                n245 = call "ICM Close Sub Panel.vi"("Queue"=w448) -> ("error out"=w447:errorcluster)  [unwired: 9 in, 1 out]
              }
            }
            n246 = property on="Scaling" class="Ring (strict)"(error in=w438) -> (error out=w440:errorcluster, "RingText.Text"=w439:string)  [unwired: 1 in, 1 out]
            n247 = invoke on="Scaling" class="SubPnl" method="Remove VI"(error in=w429) -> (error out=w428:errorcluster)  [unwired: 2 in, 2 out]
            n248 = Build Path(base path=w446, name or relative path=w439) -> (appended path=w445:path)
            n249 = Build Path(base path=w445, name or relative path="Edit Config.vi") -> (appended path=w443:path)
            n250 = Open VI Reference(vi path=w443, error in (no error)=w440) -> (vi reference=w425:refnum<vi>, error out=w426:errorcluster)  [unwired: 4 in]
            n251 = invoke class="VI" method="Run VI"(reference=w425, error in=w426, "Wait until done"=FALSE ("Wait Until Done"), "Auto Dispose Ref"=TRUE ("Auto Dispose Reference")) -> (reference out=w437:refnum<vi>, error out=w436:errorcluster)  [unwired: 1 in, 3 out]
            n252 = invoke on="Scaling" class="SubPnl" method="Insert VI"(error in=w436, "VI Ref"=w437) -> (error out=w435:errorcluster)  [unwired: 2 in, 3 out]
          }
        }
        n253 = property on="Instance" class="Ring (strict)"(error in=w416, "Strings []"=w400) -> (error out=w401:errorcluster)  [unwired: 1 in, 1 out]
        n254 = Select(t=w401, s=w401, f=w413) -> (s? t:f=w412:errorcluster)
      }
      frame "Load Output" {
      }
      frame "Error" {
        n255 = property on="Tab" class="TabCtl (strict)"() -> ("Pages"=w454:refnum<vi>[])  [unwired: 2 in, 2 out]
        n256 = local write "Tab"(ICM_Editor_Tab."Error" ("Tab")) -> ()
        n257 = for {
          tunnel: w454 -> [w465] mode=indexing
          n258 = property class="Page"(reference=w465) -> (reference out=w462:refnum<vi>, "PageLabel"=w464:string)  [unwired: 1 in, 1 out]
          n259 = Equal?(x=w464, y="Error") -> (x = y?=w459:bool)
          n260 = Select(t=T7."Page Enabled" ("Page Enabled State"), s=w459, f=T7."Page Disabled & Grayed" ("Page Enabled State")) -> (s? t:f=w461:T7)
          n261 = property class="Page"(reference=w462, "PageEnb"=w461) -> ()  [unwired: 1 in, 2 out]
        }
        "Error" <- w457
      }
      frame "Stop" {
        n262 = Unbundle By Name(w486) -> ("Parser Queue"=w485:refnum<queue>, "Bus Queue"=w482:refnum<queue>, "Scaling Queue"=w477:refnum<queue>, "Query Queue"=w476:refnum<queue>, "Config Queue"=w468:refnum<queue>)
        n263 = call "ICM Close Sub Panel.vi"("Queue"=w485) -> ("error out"=w483:errorcluster, "Queue Out"=w484:refnum<queue>)  [unwired: 9 in]
        n264 = call "ICM Close Sub Panel.vi"("Queue"=w482) -> ("error out"=w480:errorcluster, "Queue Out"=w481:refnum<queue>)  [unwired: 9 in]
        n265 = call "ICM Close Sub Panel.vi"("Queue"=w477) -> ("error out"=w479:errorcluster, "Queue Out"=w478:refnum<queue>)  [unwired: 9 in]
        n266 = call "ICM Close Sub Panel.vi"("Queue"=w476) -> ("error out"=w474:errorcluster, "Queue Out"=w475:refnum<queue>)  [unwired: 9 in]
        n267 = Release Queue(queue=w484, error in (no error)=w483) -> (error out=w473:errorcluster)  [unwired: 1 in, 2 out]
        n268 = Release Queue(queue=w481, error in (no error)=w480) -> (error out=w472:errorcluster)  [unwired: 1 in, 2 out]
        n269 = Release Queue(queue=w478, error in (no error)=w479) -> (error out=w471:errorcluster)  [unwired: 1 in, 2 out]
        n270 = Release Queue(queue=w475, error in (no error)=w474) -> (error out=w470:errorcluster)  [unwired: 1 in, 2 out]
        n271 = Release Queue(queue=w468) -> (error out=w469:errorcluster)  [unwired: 2 in, 2 out]
        n272 = flat-sequence {
          tunnel: w473 -> [_]
          tunnel: w472 -> [_]
          tunnel: w471 -> [_]
          tunnel: w470 -> [_]
          tunnel: w469 -> [_]
          frame #0 {
          }
        }
        n273 = local write "Tab"(ICM_Editor_Tab."General" ("Tab")) -> ()
        n274 = global write "ICM Editor Stop.vi" "Stop"(FALSE ("Stop")) -> ()
      }
    }
  }
